vi "Write Form Server Configuration.vi"(8 "error in (no error)":errorcluster, 10 "Form Server Configuration.lvlib:Form Server Configuration.lvclass":refnum<class "Form Server Configuration.lvclass">, 11 "Form Server in":refnum<class "Form Server.lvclass">) -> (0 "error out":errorcluster, 3 "Form Server out":refnum<class "Form Server.lvclass">)   [LabVIEW 2020, in "Form Server.lvlib" / "Form Server.lvclass"]
uses:
  Form Server.lvclass
  Form Server Configuration/Form Server Configuration.lvclass
  Form Server.lvclass/Form Server.ctl
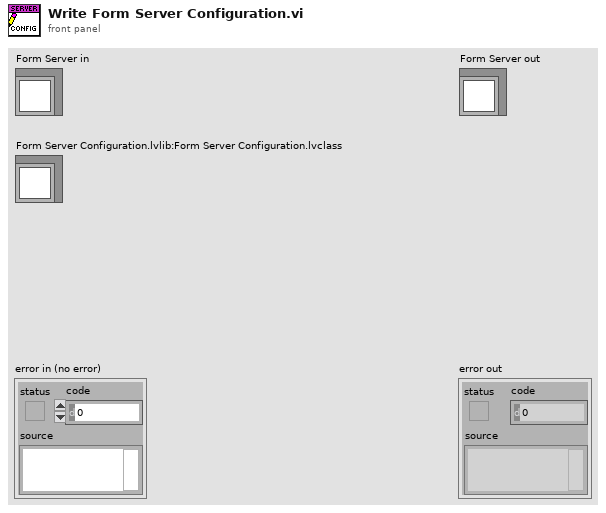
[diagram p1: front panel]
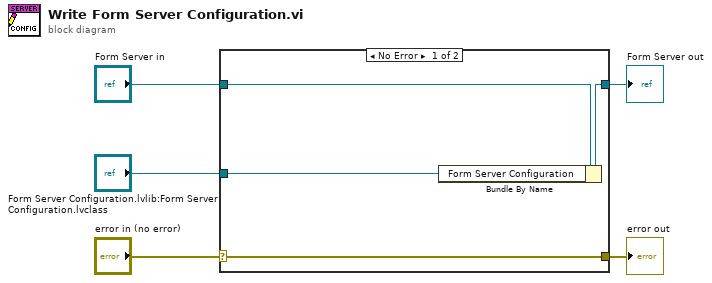
[diagram p0: block diagram]
diagram:
  n1 = case shown="No Error" "error in (no error)" {
    selector: "error in (no error)" -> [w9 w10]
    tunnel: [w9 w10] -> w4
    tunnel: [w7 w11] -> w2
    tunnel: "Form Server in" -> [w8 w11]
    tunnel: "Form Server Configuration.lvlib:Form Server Configuration.lvclass" -> [w6 _]
    frame No Error {
      n2 = Bundle By Name(cluster=w8, "Form Server Configuration"=w6) -> (w7:refnum<class "Form Server.lvclass">)
    }
    frame Error {
    }
  }
  "error out" <- w4
  "Form Server out" <- w2
